vi "Xsquared Driver Control.vi"(10 "joystick input":dbl) -> (2 "x*y":dbl)   [LabVIEW 2012]
uses:
  Robot Global Data.vi
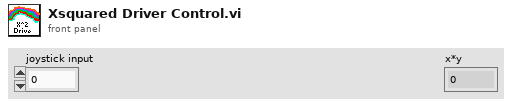
[diagram p1: front panel]
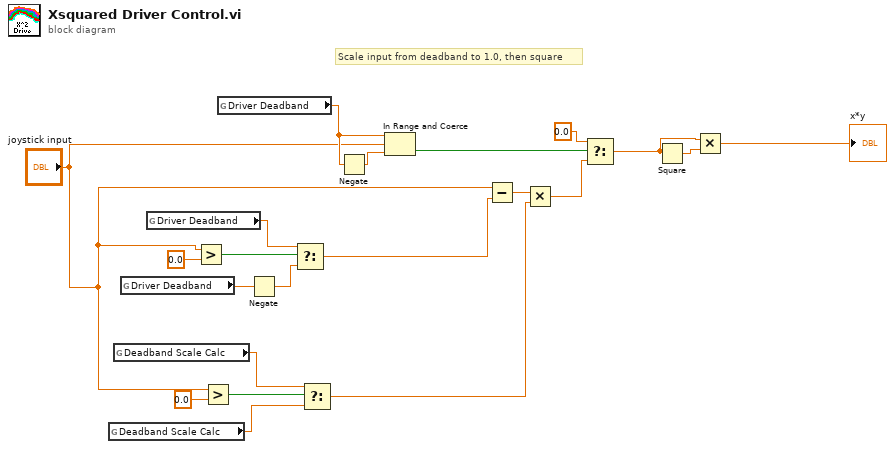
[diagram p0: block diagram]
diagram:
  # "Scale input from deadband to 1.0, then square"
  n1 = global read "Robot Global Data.vi" "Deadband Scale Calc"() -> (w2:dbl)
  n2 = global read "Robot Global Data.vi" "Deadband Scale Calc"() -> (w11:dbl)
  n3 = global read "Robot Global Data.vi" "Driver Deadband"() -> (w5:dbl)
  n4 = global read "Robot Global Data.vi" "Driver Deadband"() -> (w6:dbl)
  n5 = Greater?(x="joystick input", y=0.0) -> (0:w8:bool)
  n6 = Greater?(x="joystick input", y=0.0) -> (0:w12:bool)
  n7 = global read "Robot Global Data.vi" "Driver Deadband"() -> (w14:dbl)
  n8 = Negate(x=w5) -> (-x=w4:dbl)
  n9 = Select(t=w6, s=w8, f=w4) -> (s? t:f=w3:dbl)
  n10 = Select(t=w11, s=w12, f=w2) -> (s? t:f=w10:dbl)
  n11 = Negate(x=w14) -> (-x=w21:dbl)
  n12 = In Range and Coerce(upper limit=w14, x="joystick input", lower limit=w21) -> (In Range?=w20:bool)  [unwired: 1 out]
  n13 = Subtract(x="joystick input", y=w3) -> (x-y=w18:dbl)
  n14 = Multiply(x=w18, y=w10) -> (x*y=w17:dbl)
  n15 = Select(t=0.0, s=w20, f=w17) -> (s? t:f=w1:dbl)
  n16 = Square(x=w1) -> (x^2=w16:dbl)
  n17 = Multiply(x=w1, y=w16) -> (x*y=→"x*y":dbl)
